vi "Format Header.vi"(5 "Name":string[](array[string]), 7 "Value":string[](array[string]), 11 "JSON in":refnum<class "JSON.lvclass">) -> (3 "JSON out":refnum<class "JSON.lvclass">, 4 "Header":string)   [LabVIEW 2019, in "JSON.lvlib" / "JSON.lvclass"]
uses:
  <vilib>/gpm_packages/@cs/persistence/source/JSON/JSON.lvclass
  <vilib>/JDP Science/JSONtext/JSONtext.lvlib
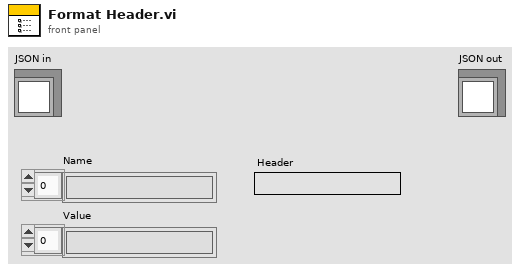
[diagram p1: front panel]
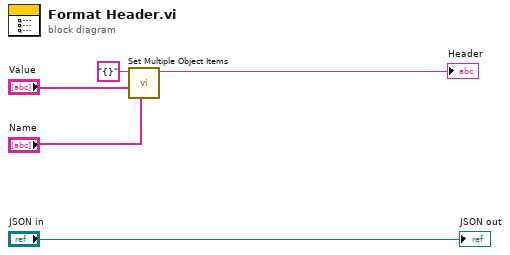
[diagram p0: block diagram]
diagram:
  n1 = call <vilib>:"Set Multiple Object Items.vi"("Item Names"="Name", "JSON Items"="Value", "JSON"="{}") -> ("<JSON>"=→"Header":string)  [unwired: 6 in, 1 out]
  "JSON out" <- "JSON in"
